vi "Add Available Measurement.vi"(8 "error in (no error)":errorcluster, 10 "Measurement.lvclass":refnum<class "Measurement.lvclass">, 11 "Controller in":refnum<class "Controller.lvclass">) -> (0 "error out":errorcluster, 3 "Controller out":refnum<class "Controller.lvclass">)   [LabVIEW 2015, in "Controller Actor.lvlib" / "Controller.lvclass"]
uses:
  Controller.lvclass
  Measurement Actor/Measurement.lvclass
  <vilib>/ActorFramework/Actor/Actor.lvclass/Actor.ctl
  <vilib>/ActorFramework/Message Enqueuer/Message Enqueuer.lvclass/Message Enqueuer.ctl
  <vilib>/ActorFramework/Message Enqueuer/Init from Existing Queue.vi
  <vilib>/ActorFramework/Message Enqueuer/Message Enqueuer.lvclass
  Messages/Log Status/Log Status.lvclass
  <vilib>/ActorFramework/Actor/Actor.lvclass
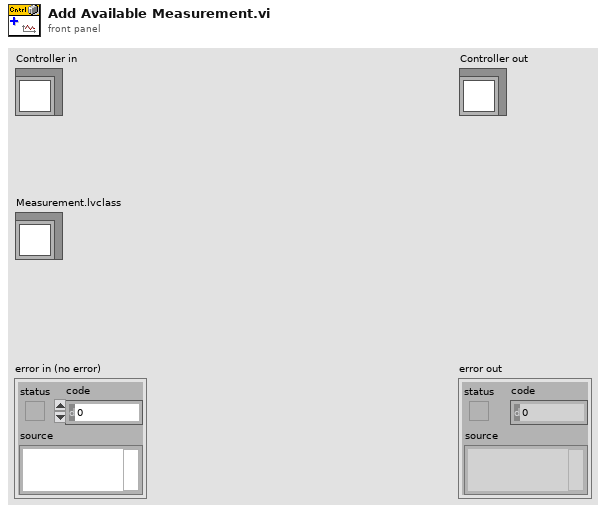
[diagram p1: front panel]
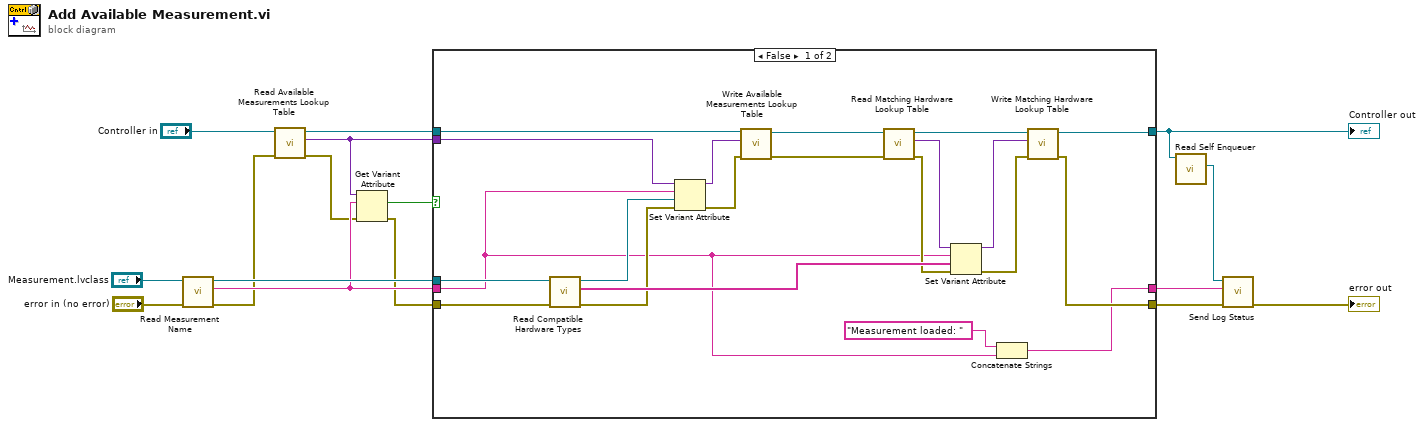
[diagram p0: block diagram]
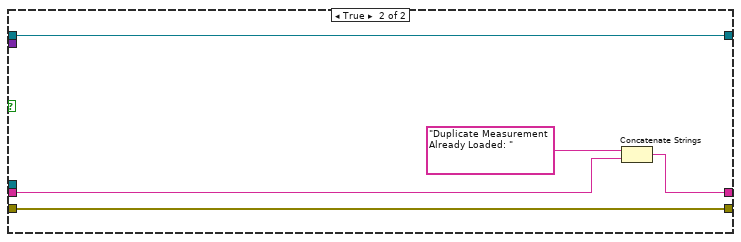
[diagram p2: hidden frame]
diagram:
  n1 = call "Read Measurement Name.vi"("error in (no error)"="error in (no error)", "Measurement in"="Measurement.lvclass") -> ("error out"=w7:errorcluster, "Measurement Name"=w8:string, "Measurement out"=w12:refnum<class "Measurement.lvclass">)  [unwired: 7 in]
  n2 = call "Read Available Measurements Lookup Table.vi"("error in (no error)"=w7, "Controller in"="Controller in") -> ("error out"=w6:errorcluster, "Available Measurements Lookup Table"=w4:variant, "Controller out"=w10:refnum<class "Controller.lvclass">)  [unwired: 7 in]
  n3 = Get Variant Attribute(Variant=w4, name=w8, error in=w6) -> (found=w9:bool, error out=w5:errorcluster)  [unwired: 1 in, 2 out]
  n4 = case shown="False" w9 {
    tunnel: [w17 w39] -> w15
    tunnel: [w22 w41] -> w2
    tunnel: w10 -> [w36 w41]
    tunnel: w12 -> [w35 _]
    tunnel: w5 -> [w20 w39]
    tunnel: w8 -> [w19 w38]
    tunnel: w4 -> [w18 _]
    tunnel: [w16 w37] -> w1
    frame False {
      n5 = call-dynamic "Read Compatible Hardware Types.vi"("error in (no error)"=w20, "Measurement in"=w35) -> ("error out"=w27:errorcluster, "Compatible Hardware Types"=w33:string[], "Measurement out"=w28:refnum<class "Measurement.lvclass">)  [unwired: 7 in]
      n6 = Set Variant Attribute(Variant=w18, name=w19, value=w28, error in=w27) -> (Variant out=w34:variant, error out=w26:errorcluster)  [unwired: 1 out]
      n7 = call "Write Available Measurements Lookup Table.vi"("error in (no error)"=w26, "Available Measurements Lookup Table"=w34, "Controller in"=w36) -> ("error out"=w25:errorcluster, "Controller out"=w30:refnum<class "Controller.lvclass">)  [unwired: 7 in]
      n8 = call "Read Matching Hardware Lookup Table.vi"("error in (no error)"=w25, "Controller in"=w30) -> ("error out"=w24:errorcluster, "Matching Hardware Lookup Table"=w32:variant, "Controller out"=w31:refnum<class "Controller.lvclass">)  [unwired: 7 in]
      n9 = Set Variant Attribute(Variant=w32, name=w19, value=w33, error in=w24) -> (Variant out=w29:variant, error out=w23:errorcluster)  [unwired: 1 out]
      n10 = Concatenate Strings("Measurement loaded: " ("string"), w19) -> (w16:string)
      n11 = call "Write Matching Hardware Lookup Table.vi"("error in (no error)"=w23, "Matching Hardware Lookup Table"=w29, "Controller in"=w31) -> ("error out"=w17:errorcluster, "Controller out"=w22:refnum<class "Controller.lvclass">)  [unwired: 7 in]
    }
    frame True {
      n12 = Concatenate Strings("Duplicate Measurement Already Loaded: " ("string"), w38) -> (w37:string)
    }
  }
  "error out" <- w15
  "Controller out" <- w2
  n13 = call <vilib>:"Read Self Enqueuer.vi"("Actor"=w2) -> ("Self Enqueuer"=w3:refnum<class "Message Enqueuer.lvclass">)  [unwired: 10 in]
  n14 = call "Send Log Status.vi"("String"=w1, "Message Enqueuer in"=w3) -> ()  [unwired: 8 in, 2 out]
